vi "Arduino_Thermistor_configure.vi"() -> ()   [LabVIEW 2013]
uses:
  Instrument drivers/Arduino/ctls_and_globals/Arduino tx msg cluster.ctl
panel:
  in  "Self-calibration interval (minutes)":sgl=1.0
  out "Output":dbl
  out "Status comment":string
  in  "Port":refnum<visa-resource-name>="COM18"
  in  "Address":u8=10
  # "Use this vi to configure the ADC self-calibration time interval\nThis value is retained in EEPROM and recalled on power-up."
  # "(255 minutes max.)\nSet 0 for never."
  # "PN 04/02/2014"
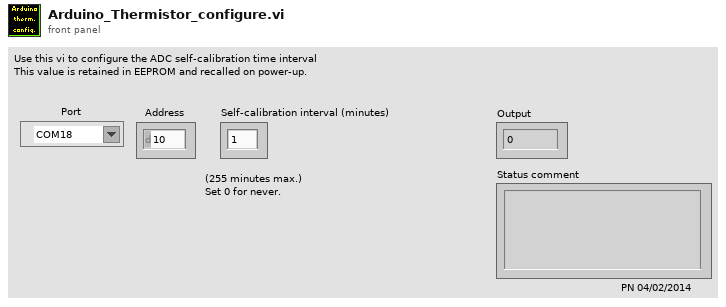
[diagram p1: front panel]
types:
  T1 = typedef "Arduino tx msg cluster.ctl" = cluster{"dest":u8, "A/D/C":string, "R/W":string, "chan":u8, "val (float)":sgl}
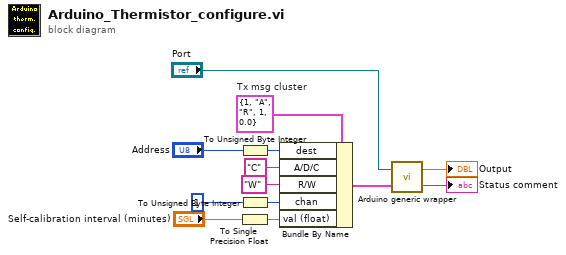
[diagram p0: block diagram]
diagram:
  w9 = T1 {"dest"=1, "A/D/C"="A", "R/W"="R", "chan"=1, "val (float)"=0.0}  # Tx msg cluster
  n1 = To Unsigned Byte Integer(number="Address") -> (unsigned 8bit integer=w6:u8)
  n2 = To Unsigned Byte Integer(number=u8 1) -> (unsigned 8bit integer=w2:u8)
  n3 = To Single Precision Float(number="Self-calibration interval (minutes)") -> (single precision float=w11:sgl)
  n4 = Bundle By Name(cluster=w9, "dest"=w6, "A/D/C"="C" ("A/D"), "R/W"="W", "chan"=w2, "val (float)"=w11) -> (w8:T1)
  n5 = call "Arduino generic wrapper.vi"("Tx msg cluster"=w8, "Port name"="Port") -> ("Scan comment"=→"Status comment":string, "Output"=→"Output":dbl)
